vi "GetDataTangent.vi"(10 "input data":string) -> (2 "tangent":dbl)   [LabVIEW 2012]
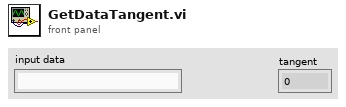
[diagram p1: front panel]
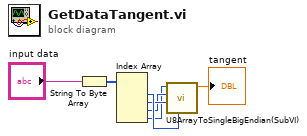
[diagram p0: block diagram]
diagram:
  n1 = String To Byte Array(string="input data") -> (unsigned byte array=w6:u8[])
  n2 = Index Array(array=w6) -> (element #1=w5:u8, element #2=w4:u8, element #3=w3:u8, element #4=w2:u8)  [unwired: 4 in]
  n3 = call "U8ArrayToSingleBigEndian(SubVI).vi"("Numeric 5"=w5, "Numeric 4"=w4, "Numeric 3"=w3, "Numeric in"=w2) -> ("Numeric 8"=→"tangent":sgl)  [unwired: 7 in]
